vi "SetBTimer.vi"(8 "error in (no error)":errorcluster) -> (0 "error out":errorcluster)   [LabVIEW 2015, in "ESLSCDLL.lvlib"]
uses:
  ESLSCDLL.lvlib
  Globals.vi
  ESLSCDLL.dll
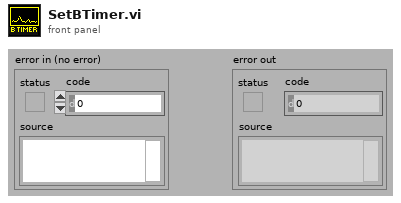
[diagram p1: front panel]
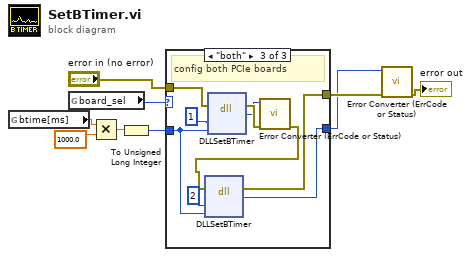
[diagram p0: block diagram]
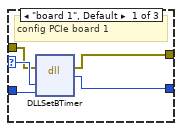
[diagram p2: hidden frame]
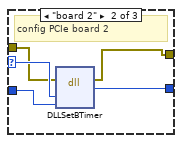
[diagram p3: hidden frame]
diagram:
  n1 = global read "Globals.vi" "btime[ms]"() -> (w2:dbl)
  n2 = global read "Globals.vi" "board_sel"() -> (w5:enum32{"0", "board 1", "board 2", "both"})
  n3 = Multiply(x=w2, y=1000.0) -> (x*y=w3:dbl)
  n4 = To Unsigned Long Integer(number=w3) -> (unsigned 32bit integer=w1:u32)
  n5 = case shown="\"both\"" w5 {
    selector: w5 -> [w14 w19 _]
    tunnel: w1 -> [w13 w18 w26]
    tunnel: [w12 w16 w21] -> w8
    tunnel: "error in (no error)" -> [w11 w17 w23]
    tunnel: [w10 w15 w20] -> w6
    frame "board 1", Default {
      # "config PCIe board 1"
      n6 = dll-call lib="C:/ENTW/PCIE/LV64/board.vis/ESLSCDLL.dll" fn="DLLSetBTimer" ("lwlscdll.dll:DLLSetTemp")(error in=w11, "drv"=w14, "btime_in_microseconds"=w13) -> (error out=w12:errorcluster, "es_status_codes"=w10:i32)  [unwired: 4 in, 1 out]
    }
    frame "board 2" {
      # "config PCIe board 2"
      n7 = dll-call lib="C:/ENTW/PCIE/LV64/board.vis/ESLSCDLL.dll" fn="DLLSetBTimer" ("lwlscdll.dll:DLLSetTemp")(error in=w17, "drv"=w19, "btime_in_microseconds"=w18) -> (error out=w16:errorcluster, "es_status_codes"=w15:i32)  [unwired: 4 in, 1 out]
    }
    frame "both" {
      # "config both PCIe boards"
      n8 = dll-call lib="C:/ENTW/PCIE/LV64/board.vis/ESLSCDLL.dll" fn="DLLSetBTimer" ("lwlscdll.dll:DLLSetTemp")(error in=w23, "drv"=u32 1, "btime_in_microseconds"=w26) -> (error out=w25:errorcluster, "es_status_codes"=w24:i32)  [unwired: 4 in, 1 out]
      n9 = call "Error Converter (ErrCode or Status).vi"("error in (no error)"=w25, "error code"=w24) -> ("error out"=w22:errorcluster)  [unwired: 9 in]
      n10 = dll-call lib="C:/ENTW/PCIE/LV64/board.vis/ESLSCDLL.dll" fn="DLLSetBTimer" ("lwlscdll.dll:DLLSetTemp")(error in=w22, "drv"=u32 2, "btime_in_microseconds"=w26) -> (error out=w21:errorcluster, "es_status_codes"=w20:i32)  [unwired: 4 in, 1 out]
    }
  }
  n11 = call "Error Converter (ErrCode or Status).vi"("error in (no error)"=w8, "error code"=w6) -> ("error out"=→"error out":errorcluster)  [unwired: 9 in]
